vi "CC Create Script Q.vi"(8 "error in (no error)":errorcluster) -> (0 "error out":errorcluster, 3 "Script Q":refnum<queue>)   [LabVIEW 2024]
uses:
  Subsystems/SS typedef cluster Instrument Command Queue Data.ctl
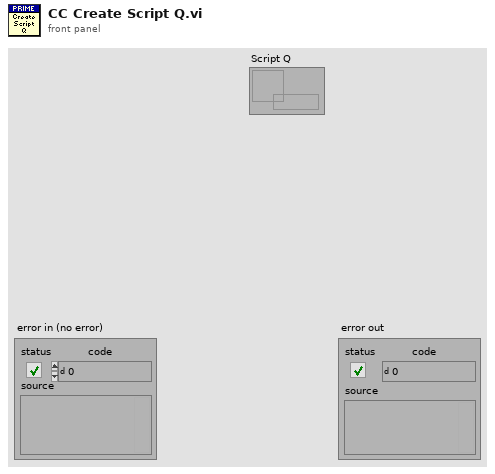
[diagram p1: front panel]
types:
  T1 = typedef "SS typedef cluster Instrument Command Queue Data.ctl" = cluster{"Cmd":string, "Parameters":variant}
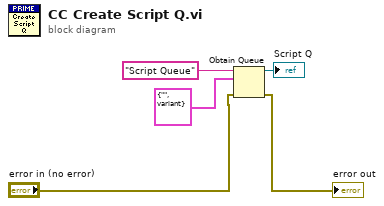
[diagram p0: block diagram]
diagram:
  n1 = Obtain Queue(name (unnamed)="Script Queue", element data type=T1 {"Cmd"="", "Parameters"=variant}, error in (no error)="error in (no error)") -> (queue out=→"Script Q":refnum<queue>, error out=→"error out":errorcluster)  [unwired: 2 in, 1 out]
